vi "Train Wheel PtByPt - DFD.vi"() -> ()   [LabVIEW 2023]
doc: "Demonstrates a simulated real-world point-by-point application. This example detects train wheel defects based on simulated real-time data acquisition and analysis.\n\nEach train has 6 wheels, and each wheel is represented by a spike in the Simulated Data chart. The height of the spike determines whether the wheel is good. After each train passes, the Bad/Good Wheels bar graph shows how good each wheel is. \n\nThe example uses VIs in the LabVIEW Digital Filter Design Toolkit to process the data."
uses:
  <vilib>/addons/Digital Filter Design/Process.llb/DFD Filtering (PtByPt).vi
  <vilib>/ptbypt/NI_PtbyPt.lvlib
  <vilib>/addons/Digital Filter Design/NI_DigFilterLicensed.lvlib
panel:
  out "Simulated Data (8 trains)":dbl(graph)=-0.7894287109375
  out "no. of wheel":u32
  in  "stop":bool
  out "Bad/Good Wheels":dbl[](graph) caption="Bad/Good Wheels (the smaller a bar the better the quality)"
  in  "fh":dbl=0.25 format="%0.4f"
  in  "threshold":dbl=15.0 format="%0.2f"
  out "no. of train":u32
  in  "length":i32=100
  in  "fl":dbl=0.01 format="%0.4f"
  in  "order":i32=4
  # "Filter Parameters"
  # "Other Parameters"
  # "Select Help»Show Context Help and move the cursor over the VI icon for more information."
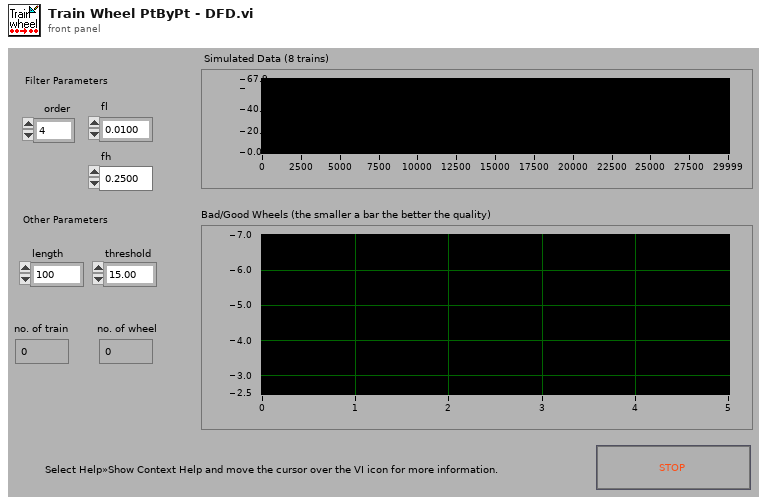
[diagram p1: front panel]
types:
  T1 = enum16{"Lowpass", "Highpass", "Bandpass", "Bandstop"}
  T2 = typedef "NI_DigFilterLicensed.lvlib/DFD Filter Obj.ctl" = cluster{"mSRate_Fs":dbl, "mSRate_Version":string, "mSRate_Comments":string, "mSRate_OrgCoef":T3, "mSRate_CurCoef":T3, "mSRate_Quantized?":bool, "mSRate_QCoef":T3, "mSRate_QSettings":T5[], "mSRate_Order":i32, "mSRate_Scaling":cluster{"mSRate_ScaleByPowerOf2?":bool, "mSRate_ScaleType":T7}}
  T3 = typedef "NI_DigFilterLicensed.lvlib/DFD Filter Coef.ctl" = cluster{"type":T4, "gain":dbl, "coef a (k)":dbl[], "coef b (v)":dbl[]}
  T4 = typedef "NI_DigFilterLicensed.lvlib/DFD Filter Structure Type Selector.ctl" = enum16{"Undefined", "FIR Direct Form", "FIR Direct Form Transposed", "FIR Symmetric", "FIR Antisymmetric", "IIR Direct Form I", "IIR Direct Form I Transposed", "IIR Direct Form II", "IIR Direct Form II Transposed", "IIR Cascaded Second Order Sections Form I", "IIR Cascaded Second Order Sections Form I Transposed", "IIR Cascaded Second Order Sections Form II", "IIR Cascaded Second Order Sections Form II Transposed", "Lattice Allpass (basic sections)", "Lattice Allpass (one multiplier sections)", "Lattice Allpass (normalized sections)", "Lattice AR (basic sections)", "Lattice AR (one multiplier sections)", "Lattice AR (normalized sections)", "Lattice MA (minimum phase)", "Lattice MA (maximum phase)", "Lattice ARMA (basic sections)", "Lattice ARMA (one multiplier sections)", "Lattice ARMA (normalized sections)"}
  T5 = typedef "NI_DigFilterLicensed.lvlib/dfd_Internal Quantization Settings.ctl" = cluster{"source":T6, "wl":i16, "iwl":i16, "overflow mode":enum16{"Saturation", "Wrap"}, "rounding mode":enum16{"Nearest", "Truncation"}, "signed?":bool}
  T6 = typedef "NI_DigFilterLicensed.lvlib/dfd_Internal Quantization Srcs.ctl" = u16
  T7 = typedef "NI_DigFilterLicensed.lvlib/DFD Coef Norm Type.ctl" = enum16{"No Norm", "Time Domain 1-Norm", "Time Domain 2-Norm", "Time Domain Inf-Norm"}
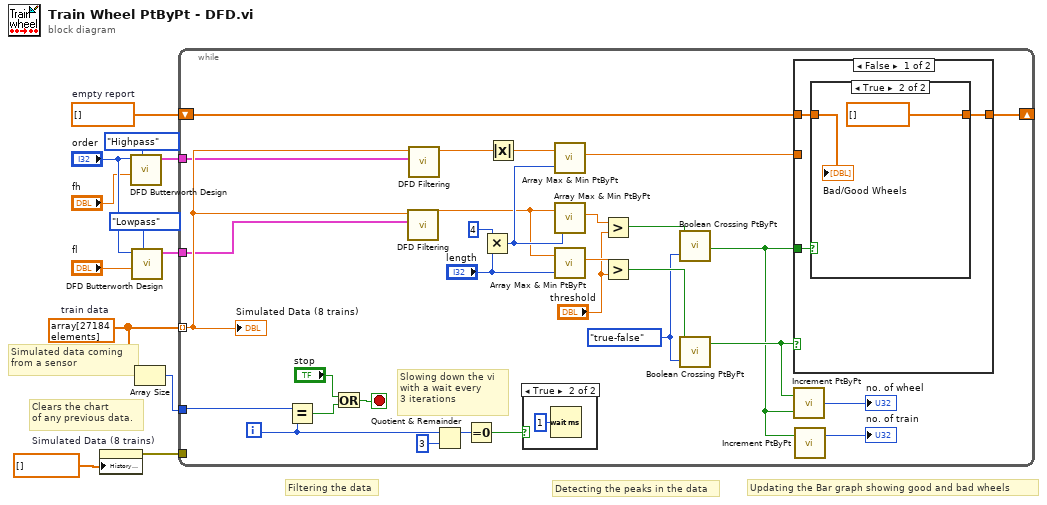
[diagram p0: block diagram]
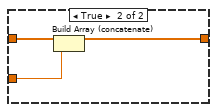
[diagram p4: hidden frame]
diagram:
  w8 = dbl[] array[27184 elements]  # train data
  w12 = dbl[] []  # empty report
  # "Updating the Bar graph showing good and bad wheels"
  # "Detecting the peaks in the data"
  # "Filtering the data"
  # "Clears the chart \nof any previous data."
  # "Simulated data coming \nfrom a sensor"
  n1 = property on="Simulated Data (8 trains)" class="WFChart (strict)"("History Data"=dbl[] []) -> (error out=w10:errorcluster)  [unwired: 2 in, 1 out]
  n2 = call <vilib>:"DFD Butterworth Design.vi"("filter type"=T1."Highpass", "low cutoff freq [Hz]"="fh", "order"="order") -> ("filter out"=w2:T2)  [unwired: 3 in, 5 out]
  n3 = call <vilib>:"DFD Butterworth Design.vi"("filter type"=T1."Lowpass", "low cutoff freq [Hz]"="fl", "order"="order") -> ("filter out"=w1:T2)  [unwired: 3 in, 5 out]
  n4 = Array Size(array=w8) -> (size(s)=w9:i32)
  n5 = while {
    shift-left: w12 -> [w36]
    shift-right: [w37] -> _
    tunnel: w8 -> [w16] mode=indexing
    tunnel: w10 -> [_]
    tunnel: w9 -> [w25]
    tunnel: w2 -> [w14]
    tunnel: w1 -> [w13]
    i -> [w24]
    stop <- w28 stop-if-true
    w18 = enum16{"either", "false-true", "true-false"}."true-false" ("direction")
    # "Slowing down the vi\nwith a wait every \n3 iterations"
    n6 = Equal?(x=w25, y=w24) -> (x = y?=w19:bool)
    n7 = Or(x="stop", y=w19) -> (x .or. y?=w28:bool)
    n8 = call-poly <vilib>:"DFD Filtering.vi"("filter"=w13, "signal in"=w16) -> ("signal out"=w15:dbl)  [unwired: 2 in, 7 out]
    n9 = call-poly <vilib>:"DFD Filtering.vi"("filter"=w14, "signal in"=w16) -> ("signal out"=w17:dbl)  [unwired: 2 in, 7 out]
    n10 = Quotient & Remainder(x=w24, y=3) -> (x-y*floor(x/y)=w22:i32)  [unwired: 1 out]
    n11 = Equal To 0?(x=w22) -> (x = 0?=w21:bool)
    n12 = Multiply(x=4, y="length") -> (x*y=w31:i32)
    n13 = Absolute Value(x=w17) -> (abs(x)=w38:dbl)
    n14 = case shown="True" w21 {
      frame False {
      }
      frame True {
        n15 = Wait (ms)(milliseconds to wait=u32 1) -> ()  [unwired: 1 out]
      }
    }
    n16 = call <vilib>:"Array Max & Min PtByPt.vi"("input data point"=w38, "sample length"=w31) -> ("max value"=w39:dbl)  [unwired: 1 in, 4 out]
    n17 = call <vilib>:"Array Max & Min PtByPt.vi"("input data point"=w15, "sample length"=w31) -> ("max value"=w35:dbl)  [unwired: 1 in, 4 out]
    n18 = call <vilib>:"Array Max & Min PtByPt.vi"("input data point"=w15, "sample length"="length") -> ("max value"=w42:dbl)  [unwired: 1 in, 4 out]
    n19 = Greater?(x=w35, y="threshold") -> (0:w33:bool)
    n20 = Greater?(x=w42, y="threshold") -> (0:w32:bool)
    n21 = call <vilib>:"Boolean Crossing PtByPt.vi"("direction"=w18, "input"=w33) -> ("crossing"=w26:bool)  [unwired: 1 in]
    n22 = call <vilib>:"Boolean Crossing PtByPt.vi"("direction"=w18, "input"=w32) -> ("crossing"=w27:bool)  [unwired: 1 in]
    n23 = case shown="False" w27 {
      tunnel: w39 -> [_ w50]
      tunnel: w26 -> [w46 _]
      tunnel: [w45 w51] -> w37
      tunnel: w36 -> [w44 w52]
      frame False {
        n24 = case shown="True" w46 {
          tunnel: [w47 dbl[] []] -> w45
          tunnel: w44 -> [w47 w49]
          frame False {
          }
          frame True {
            "Bad/Good Wheels" <- w49
          }
        }
      }
      frame True {
        n25 = Build Array (concatenate)(w52, w50) -> (w51:dbl[])
      }
    }
    n26 = call <vilib>:"Increment PtByPt.vi"("initialize"=w26, "activate"=w27) -> ("counter"=→"no. of wheel":u32)  [unwired: 1 out]
    n27 = call <vilib>:"Increment PtByPt.vi"("activate"=w26) -> ("counter"=→"no. of train":u32)  [unwired: 1 in, 1 out]
    "Simulated Data (8 trains)" <- w16
  }
